vi "Set Row Heights.vi"(7 "Row Heights":i32[](array[numeric]), 8 "error in (no error)":errorcluster, 10 "Sheet Reference":refnum<k24>) -> (0 "error out":errorcluster, 2 "Sheet Reference out":refnum<k24>)   [LabVIEW 2014]
uses:
  C:/PhaeronGit/LVNPOI/Resources/NPOI 2.1.1 dotnet2/NPOI.dll
  Resources/NPOI 2.1.1 dotnet2/NPOI.dll
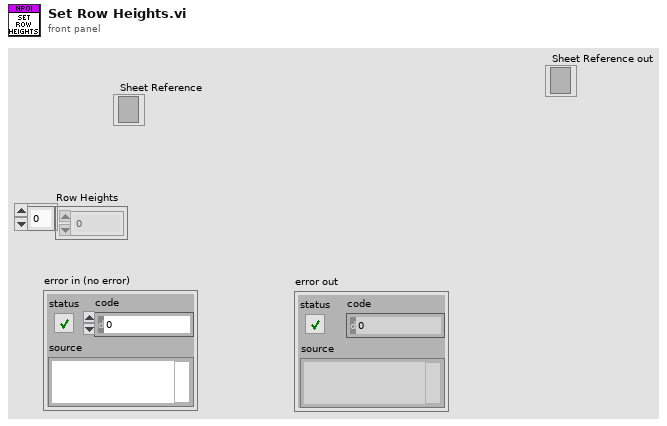
[diagram p1: front panel]
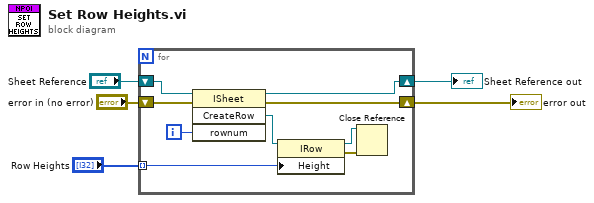
[diagram p0: block diagram]
diagram:
  n1 = for {
    shift-right: [w12] -> w2
    shift-left: "Sheet Reference" -> [w14]
    shift-right: [w11] -> w1
    shift-left: "error in (no error)" -> [w13]
    tunnel: "Row Heights" -> [w8] mode=indexing
    i -> [w10]
    n2 = invoke class="ISheet" method="CreateRow"(reference=w14, error in=w13, "rownum"=w10) -> (reference out=w12:refnum<k24>, error out=w11:errorcluster, "CreateRow"=w9:refnum<k24>)  [unwired: 1 in, 1 out]
    n3 = property class="IRow"(reference=w9, "Height"=w8) -> (reference out=w6:refnum<k24>, error out=w7:errorcluster)  [unwired: 1 in]
    n4 = Close Reference(reference=w6, error in (no error)=w7) -> ()  [unwired: 1 out]
  }
  "Sheet Reference out" <- w2
  "error out" <- w1
